vi "FromRepo.vi"(8 "error in":errorcluster, 9 "cluster":T2, 10 "repository in":refnum<class "NISE_CEF_Repository.lvclass">, 11 "SequenceNode in":refnum<class "SequenceNode.lvclass">) -> (0 "error out":errorcluster, 2 "repository out":refnum<class "NISE_CEF_Repository.lvclass">, 3 "node":T1)   [LabVIEW 2015, in "SequenceNode.lvclass"]
doc: "Copyright 2017 National Instruments Corporation\n\nLicensed under the Apache License, Version 2.0 (the \"License\"); you may not use this file except in compliance with the License. You may obtain a copy of the License at http://www.apache.org/licenses/LICENSE-2.0\nUnless required by applicable law or agreed to in writing, software distributed under the License is distributed on an \"AS IS\" BASIS, WITHOUT WARRANTIES OR CONDITIONS OF ANY KIND, either express or implied. See the License for the specific language governing permissions and limitations under the License."
uses:
  SequenceNode.lvclass
  <vilib>/NI/Configuration Framework/Repository/NISE_CEF_Repository.lvclass
  <vilib>/NI/Configuration Framework/Node/FromRepoCluster.ctl
  <vilib>/NI/Configuration Framework/Node/NodeRef.ctl
  <vilib>/NI/Configuration Framework/Node/NISE_CEF_Node.lvclass
  SequenceRepo/SequenceRepo.lvclass
  Prototype/classes/Sequence/Config/Sequence Config.lvclass
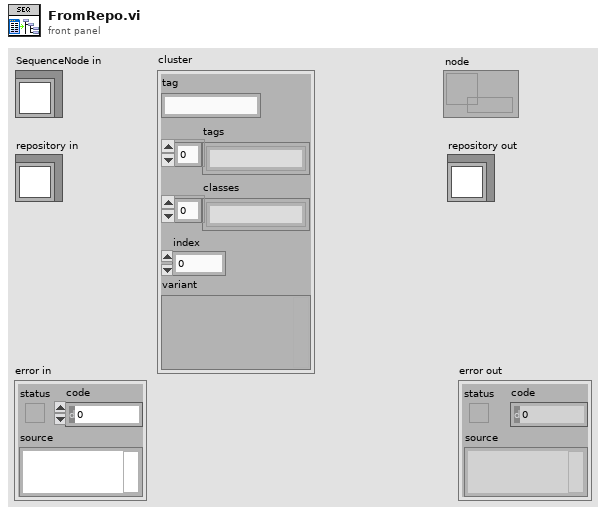
[diagram p1: front panel]
types:
  T1 = typedef "NISE_CEF_Node.lvclass/NodeRef.ctl" = refnum<data-value>
  T2 = typedef "NISE_CEF_Node.lvclass/FromRepoCluster.ctl" = cluster{"tag":string, "tags":string[], "classes":string[], "index":i32, "variant":variant}
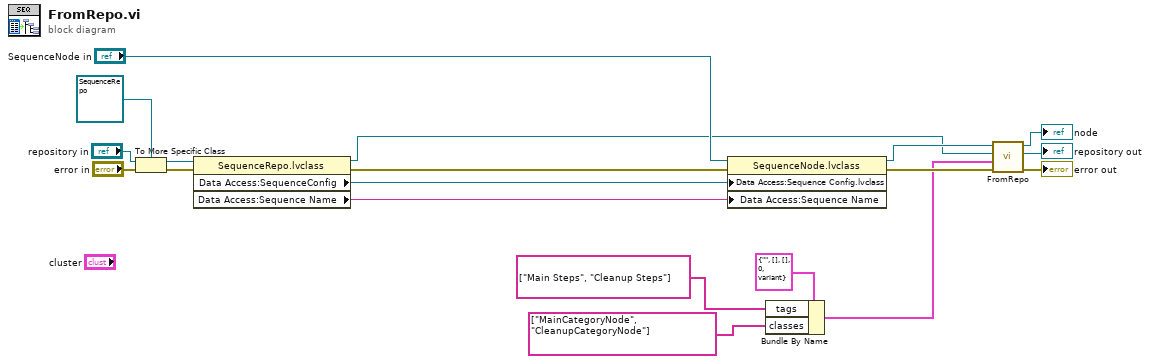
[diagram p0: block diagram]
diagram:
  n1 = To More Specific Class(target class=refnum<class "SequenceRepo.lvclass"> refnum ("cRIO repo.lvclass"), reference="repository in", error in="error in") -> (specific class reference=w13:refnum<class "SequenceRepo.lvclass">, error out=w10:errorcluster)
  n2 = property class="SequenceRepo.lvclass"(reference=w13, error in=w10) -> (reference out=w12:refnum<class "SequenceRepo.lvclass">, error out=w7:errorcluster, "Data Access:SequenceConfig"=w6:refnum<class "Sequence Config.lvclass">, "Data Access:Sequence Name"=w5:string)
  n3 = property class="SequenceNode.lvclass"(reference="SequenceNode in", error in=w7, "Data Access:Sequence Config.lvclass"=w6, "Data Access:Sequence Name"=w5) -> (reference out=w16:refnum<class "SequenceNode.lvclass">, error out=w9:errorcluster)
  n4 = Bundle By Name(cluster=T2 {"tag"="", "tags"=[], "classes"=[], "index"=0, "variant"=variant} ("from repo cluster"), "tags"=string[] ["Main Steps", "Cleanup Steps"], "classes"=string[] ["MainCategoryNode", "CleanupCategoryNode"]) -> (w3:T2)
  n5 = call-parent "FromRepo.vi"("error in"=w9, "from repo cluster"=w3, "repository in"=w12, "node in"=w16) -> ("error out"=→"error out":errorcluster, "repository out"=→"repository out":refnum<class "NISE_CEF_Repository.lvclass">, "node"=→"node":T1)  [unwired: 5 in]
